vi "String to Threshold Configuration.vi"(8 "Error In":errorcluster, 11 "String":string) -> (0 "Error Out":errorcluster, 2 "Callback Threshold":T1, 3 "rest of String":string)   [LabVIEW 2011, in "Tinkerforge.lvlib" / "Device.lvclass"]
doc: "This VI converts the binary callback threshold string to a cluster."
uses:
  Device.lvclass
  Type Definitions/Callback Threshold.ctl
  Type Definitions/Callback Option.ctl
  IP Connection/IP Connection.lvclass
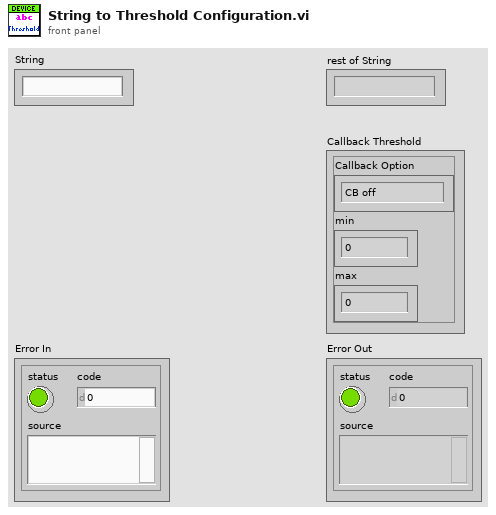
[diagram p1: front panel]
types:
  T1 = typedef "Tinkerforge.lvlib/Device.lvclass/Callback Threshold.ctl" = cluster{"Callback Option":T2, "min":i16, "max":i16}
  T2 = typedef "Tinkerforge.lvlib/Device.lvclass/Callback Option.ctl" = enum8{"CB off", "outside range", "inside range", "smaller", "greater"}
  T3 = enum16{"big-endian, network order", "native, host order", "little-endian"}
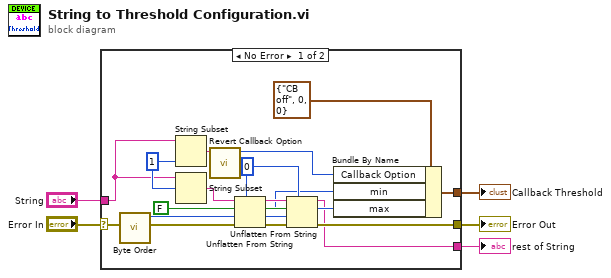
[diagram p0: block diagram]
diagram:
  n1 = case shown="No Error" "Error In" {
    selector: "Error In" -> [w17 w24]
    tunnel: "String" -> [w13 w23]
    tunnel: [w15 w24] -> w3
    tunnel: [w7 _] -> w2
    tunnel: [w6 w23] -> w1
    frame No Error {
      w20 = 1 ("length (rest)")
      w21 = i16 0
      w12 = FALSE
      n2 = call "Byte Order.vi"() -> ("byte order (2:little-endian)"=w14:T3)  [unwired: 11 in]
      n3 = String Subset(string=w13, length (rest)=w20) -> (substring=w18:string)  [unwired: 1 in]
      n4 = String Subset(string=w13, offset (0)=w20) -> (substring=w19:string)  [unwired: 1 in]
      n5 = call "Revert Callback Option.vi"("Callback Option String"=w18) -> ("Callback Option"=w8:T2)  [unwired: 10 in]
      n6 = Unflatten From String(type=w21, binary string=w19, data includes array or string size? (T)=w12, byte order (0:big-endian, network order)=w14, error in (no error)=w17) -> (rest of the binary string=w22:string, value=w9:i16, error out=w16:errorcluster)
      n7 = Unflatten From String(type=w21, binary string=w22, data includes array or string size? (T)=w12, byte order (0:big-endian, network order)=w14, error in (no error)=w16) -> (rest of the binary string=w6:string, value=w10:i16, error out=w15:errorcluster)
      n8 = Bundle By Name(cluster=T1 {"Callback Option"=enum."CB off", "min"=0, "max"=0} ("Callback Threshold"), "Callback Option"=w8, "min"=w9, "max"=w10) -> (w7:T1)
    }
    frame Error {
    }
  }
  "Error Out" <- w3
  "Callback Threshold" <- w2
  "rest of String" <- w1
